vi "UserInterface_ZA.vi"(8 "error in":errorcluster, 9 "Zen Analytics":refnum<class "Zen Analytics.lvclass">, 11 "InitializationData":refnum<user-event>) -> (0 "error out":errorcluster)   [LabVIEW 2019, in "Zen Analytics.lvlib" / "Zen Analytics.lvclass"]
uses:
  Zen Analytics.lvclass
  Dependency/GraphReff.ctl
  <vilib>/Utility/miscctls.llb/LVRowAndColumnTypeDef.ctl
  <vilib>/Utility/miscctls.llb/LVBoundsTypeDef.ctl
panel:
  out "Bar graph":dbl[][](graph) caption="Defect Summary"
  out "Yeild Chart":picture
  out "Labels":picture
  out "Measurement-Summary -1":T1(graph)={"Start"=1, "index"=0, "Waveform Graph"=[]} caption="A Summary"
  out "Histogram Summary":T2(graph) caption="A Summary"
  in  "Select Measurement":u16(ring) items=["A", "C", "D"]
  out "Cp-CpkTable":string[][](table)=[["1.13", "1.14", "1.13", "1.16", "1.18"], ["1.14", "1.12", "1.12", "1.01", "1.02"], ["1.29", "1.26", "1.26", "1.03", "1.04"], ["0.10", "0.10", "0.13", "0.13", "0.11"], ["-0.05", "-0.10", "-0.17", "-0.07", "-0.22"]]
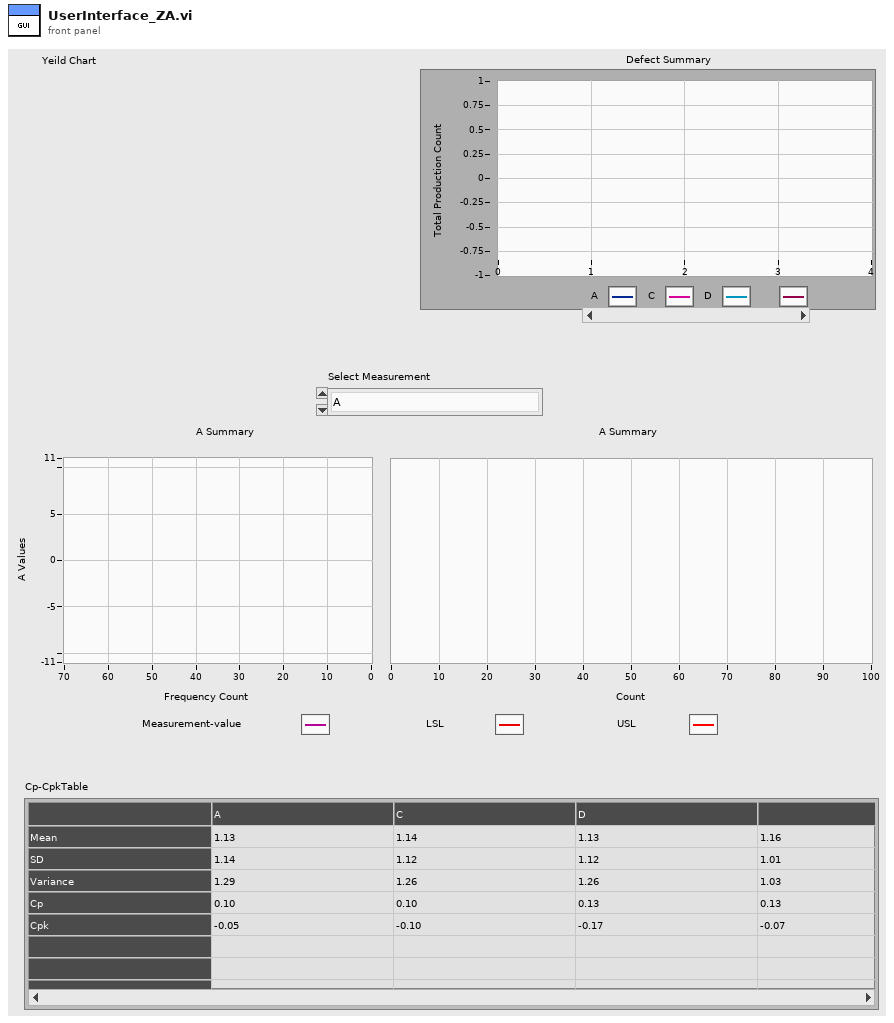
[diagram p1: front panel]
types:
  T1 = cluster{"Start":i32, "index":i32, "Waveform Graph":dbl[][]}
  T2 = cluster{"X Values":dbl[], "Best Gaussian Fit":dbl[]}[]
  T3 = typedef "LVRowAndColumnTypeDef.ctl" = cluster{"Row":i32, "Column":i32}
  T4 = typedef "LVBoundsTypeDef.ctl" = cluster{"Width":u32, "Height":u32}
  T5 = typedef "Zen Analytics.lvlib/Zen Analytics.lvclass/GraphReff.ctl" = cluster{"HistgramGraph-reff":refnum<vi>[], "BarGraph-reff":refnum<vi>[], "PieGraph-reff":refnum<vi>[], "Lable-reff":refnum<vi>[], "TrendGraph-reff":refnum<vi>[], "CpCpkTable":refnum<vi>}
  T6 = cluster{"ColumnNo":i32, "MeasurementData":cluster{"Measurement ID":i32, "Measurement Name":string, "Nominal Values":dbl, "LSL":dbl, "USL":dbl, "LCL":dbl, "UCL":dbl}[]}
  T7 = cluster{"Measurement ID":i32, "Measurement Name":string, "Nominal Values":dbl, "LSL":dbl, "USL":dbl, "LCL":dbl, "UCL":dbl}[]
  T8 = cluster{"Measurement-ID":i32[], "Measurement Names":string[], "NominalValues":dbl[], "LSL":dbl[], "USL":dbl[], "LCL":dbl[], "UCL":dbl[]}
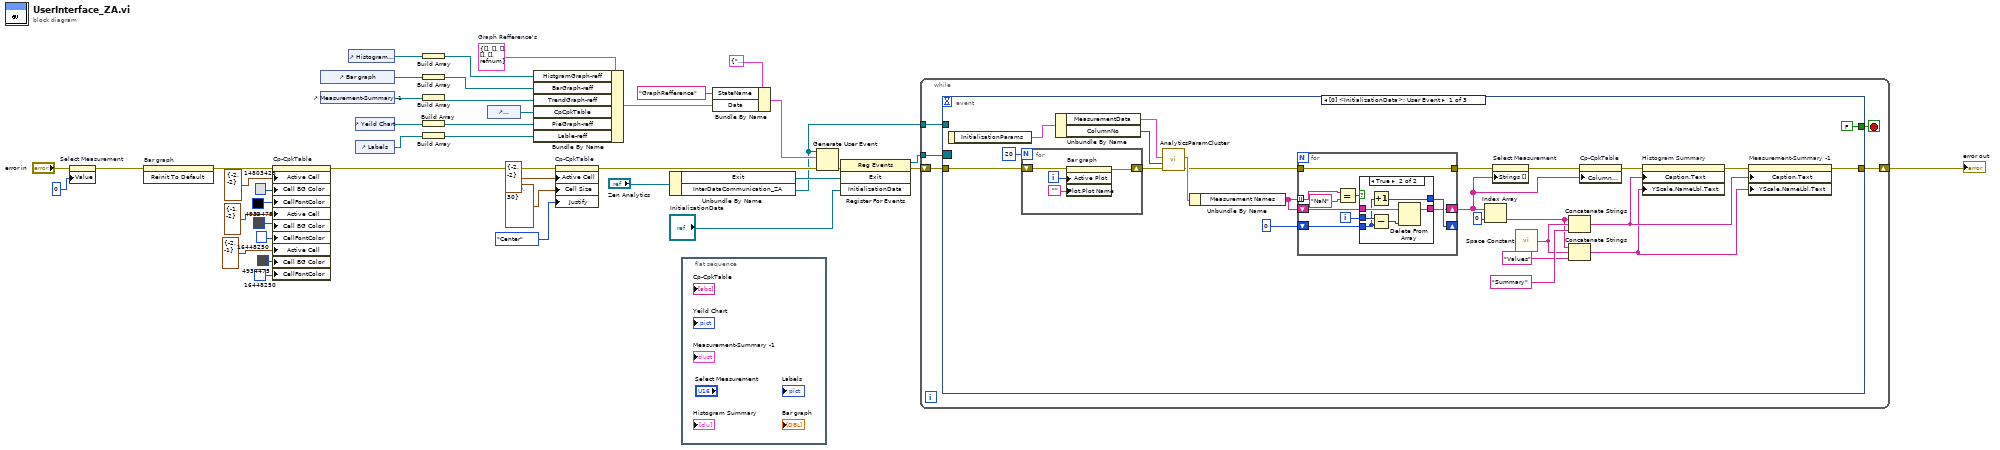
[diagram p0: block diagram]
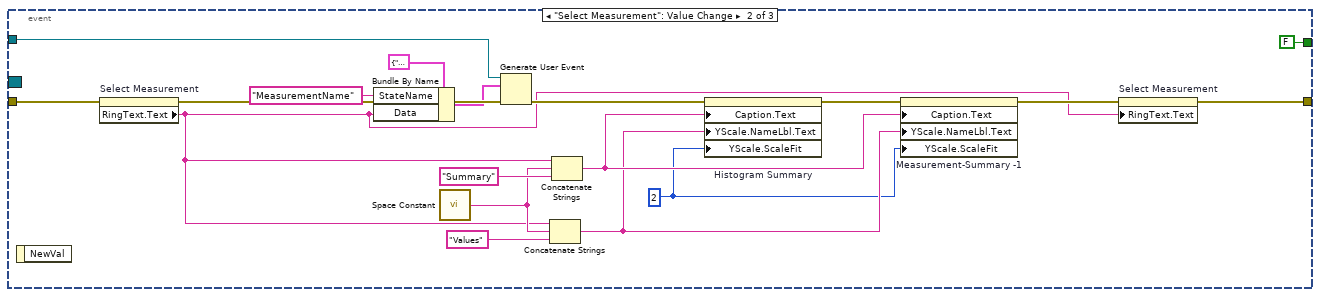
[diagram p3: hidden frame]
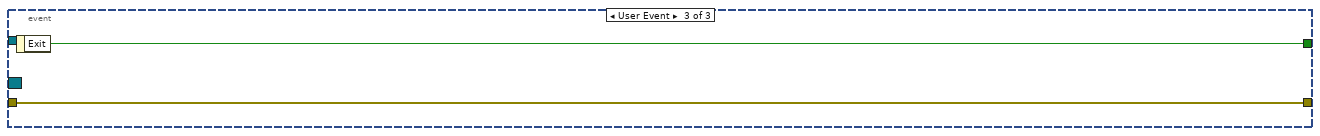
[diagram p4: hidden frame]
diagram:
  w39 = T5 {"HistgramGraph-reff"=[], "BarGraph-reff"=[], "PieGraph-reff"=[], "Lable-reff"=[], "TrendGraph-reff"=[], "CpCpkTable"=refnum}  # Graph Refference's
  n1 = property on="Select Measurement" class="Ring (strict)"(error in="error in", "Value"=0) -> (error out=w9:errorcluster)  [unwired: 1 in, 1 out]
  n2 = invoke on="Bar graph" class="WFGraph (strict)" method="Reinit To Default"(error in=w9) -> (error out=w8:errorcluster)  [unwired: 2 in, 2 out]
  n3 = property on="Cp-CpkTable" class="Tbl (strict)"(error in=w8, "Active Cell"=T3 {"Row"=-2, "Column"=-2} ("Active Cell:Active Cell"), "Cell BG Color"=u32 14803425, "CellFontColor"=u32 0, "Active Cell"=T3 {"Row"=-1, "Column"=-2} ("Active Cell:Active Cell"), "Cell BG Color"=u32 4934475, "CellFontColor"=u32 16448250, "Active Cell"=T3 {"Row"=-2, "Column"=-1} ("Active Cell:Active Cell"), "Cell BG Color"=u32 4934475, "CellFontColor"=u32 16448250) -> (error out=w24:errorcluster)  [unwired: 1 in, 1 out]
  n4 = control-ref of="Bar graph"() -> (w10:refnum<vi>)
  n5 = control-ref of="Measurement-Summary -1"() -> (w28:refnum<vi>)
  n6 = control-ref of="Histogram Summary"() -> (w27:refnum<vi>)
  n7 = control-ref of="Yeild Chart"() -> (w19:refnum<vi>)
  n8 = control-ref of="Labels"() -> (w20:refnum<vi>)
  n9 = Build Array(w27) -> (w38:refnum<vi>[])
  n10 = Build Array(w10) -> (w35:refnum<vi>[])
  n11 = Build Array(w28) -> (w37:refnum<vi>[])
  n12 = Build Array(w19) -> (w22:refnum<vi>[])
  n13 = Build Array(w20) -> (w21:refnum<vi>[])
  n14 = control-ref of="Cp-CpkTable"() -> (w36:refnum<vi>)
  n15 = Bundle By Name(cluster=w39, "HistgramGraph-reff"=w38, "BarGraph-reff"=w35, "TrendGraph-reff"=w37, "CpCpkTable"=w36, "PieGraph-reff"=w22, "Lable-reff"=w21) -> (w14:T5)
  n16 = property on="Cp-CpkTable" class="Tbl (strict)"(error in=w24, "Active Cell"=T3 {"Row"=-2, "Column"=-2} ("Active Cell:Active Cell"), "Cell Size"=T4 {"Width"=180, "Height"=30} ("Active Cell:Cell Size"), "Justify"=enum16{"Left", "Center", "Right"}."Center" ("Active Cell:Cell Justification")) -> (error out=w23:errorcluster)  [unwired: 1 in, 1 out]
  n17 = Unbundle By Name("Zen Analytics") -> ("Exit"=w31:refnum<user-event>, "InterDataCommunication_ZA"=w11:refnum<user-event>)
  n18 = flat-sequence {
    frame #0 {
    }
  }
  n19 = Bundle By Name(cluster=cluster{"StateName":string, "Data":variant} {"StateName"="", "Data"=variant} ("event data"), "StateName"="GraphRefference", "Data"=w14) -> (w15:cluster{"StateName":string, "Data":variant})
  n20 = Generate User Event(user event=w11, event data cluster=w15, error in=w23) -> (error out=w34:errorcluster)  [unwired: 1 in, 1 out]
  n21 = register-events(error in=w34, w31, "InitializationData") -> (reference out=w32:refnum<event-registration>, error out=w33:errorcluster)  [unwired: 1 in]
  n22 = while {
    shift-right: [w46] -> w25
    shift-left: w33 -> [w47]
    tunnel: w32 -> [w45]
    tunnel: w11 -> [w43]
    stop <- w44 stop-if-true
    n23 = event shown="[0] <InitializationData>: User Event" {
      selector: w45 -> [_ _ _]
      dyn-events: _ -> [_ _ _]
      timeout: _ -> [_ _ _]
      tunnel: w47 -> [w50 w110 w111]
      tunnel: [w56 w94 w111] -> w46
      tunnel: [FALSE ("Exit") FALSE ("Exit") w112] -> w44
      tunnel: w43 -> [_ w102 _]
      event User Event {
        n24 = event-data() -> ("InitializationParams"=w54:T6)  [unwired: 1 in]
        n25 = for {
          N: 20 -> [_]
          shift-right: [w72] -> w49
          shift-left: w50 -> [w73]
          i -> [w75]
          n26 = property on="Bar graph" class="WFGraph (strict)"(error in=w73, "Active Plot"=w75, "Plot.Plot Name"="") -> (error out=w72:errorcluster)  [unwired: 1 in, 1 out]
        }
        n27 = Unbundle By Name(w54) -> ("MeasurementData"=w53:T7, "ColumnNo"=w52:i32)
        n28 = call "AnalyticsParamCluster.vi"("error in (no error)"=w49, "Number of columns"=w52, "MeasurementData"=w53) -> ("error out"=w60:errorcluster, "Initialization Data"=w71:T8)  [unwired: 6 in, 1 out]
        n29 = Unbundle By Name(w71) -> ("Measurement Names"=w63:string[])
        n30 = for {
          tunnel: w63 -> [w78] mode=indexing
          shift-right: [w83] -> _
          shift-left: 0 -> [w84]
          shift-right: [w80] -> w57
          shift-left: w63 -> [w81]
          tunnel: [w76] -> w55
          tunnel: w60 -> [w76]
          i -> [w82]
          n31 = Equal?(x=w78, y="NaN") -> (x = y?=w77:bool)
          n32 = case shown="True" w77 {
            tunnel: w81 -> [w85 w92]
            tunnel: w84 -> [w86 w87]
            tunnel: [w86 w90] -> w83
            tunnel: [w85 w91] -> w80
            tunnel: w82 -> [_ w88]
            frame False {
            }
            frame True {
              n33 = Increment(x=w87) -> (x+1=w90:i32)
              n34 = Subtract(x=w88, y=w87) -> (x-y=w89:i32)
              n35 = Delete From Array(array=w92, index=w89) -> (array with subset deleted=w91:string[])  [unwired: 1 in, 1 out]
            }
          }
        }
        n36 = Index Array(array=w57, index=0) -> (element=w59:string)
        n37 = property on="Select Measurement" class="Ring (strict)"(error in=w55, "Strings []"=w57) -> (error out=w67:errorcluster)  [unwired: 1 in, 1 out]
        n38 = call <vilib>:"Space Constant.vi"() -> ("String"=w65:string)
        n39 = Concatenate Strings(w59, w65, "Summary" ("string")) -> (w68:string)
        n40 = Concatenate Strings(w59, w65, "Values" ("string")) -> (w58:string)
        n41 = property on="Cp-CpkTable" class="Tbl (strict)"(error in=w67, "Column Headers[]"=w57) -> (error out=w66:errorcluster)  [unwired: 1 in, 1 out]
        n42 = property on="Histogram Summary" class="XYGraph (strict)"(error in=w66, "Caption.Text"=w68, "YScale.NameLbl.Text"=w58) -> (error out=w69:errorcluster)  [unwired: 1 in, 1 out]
        n43 = property on="Measurement-Summary -1" class="WFGraph (strict)"(error in=w69, "Caption.Text"=w68, "YScale.NameLbl.Text"=w58) -> (error out=w56:errorcluster)  [unwired: 1 in, 1 out]
      }
      event "Select Measurement": Value Change {
        w96 = u8 2 ("Y Scale.Scale Fit")
        n44 = event-data() -> ()  [unwired: 1 in, 1 out]
        n45 = property on="Select Measurement" class="Ring (strict)"(error in=w110) -> (error out=w109:errorcluster, "RingText.Text"=w93:string)  [unwired: 1 in, 1 out]
        n46 = Bundle By Name(cluster=cluster{"StateName":string, "Data":variant} {"StateName"="", "Data"=variant} ("event data"), "StateName"="MeasurementName", "Data"=w93) -> (w99:cluster{"StateName":string, "Data":variant})
        n47 = call <vilib>:"Space Constant.vi"() -> ("String"=w98:string)
        n48 = Generate User Event(user event=w102, event data cluster=w99, error in=w109) -> (error out=w107:errorcluster)  [unwired: 1 in, 1 out]
        n49 = Concatenate Strings(w93, w98, "Values" ("string")) -> (w103:string)
        n50 = Concatenate Strings(w93, w98, "Summary" ("string")) -> (w105:string)
        n51 = property on="Histogram Summary" class="XYGraph (strict)"(error in=w107, "Caption.Text"=w105, "YScale.NameLbl.Text"=w103, "YScale.ScaleFit"=w96) -> (error out=w106:errorcluster)  [unwired: 1 in, 1 out]
        n52 = property on="Measurement-Summary -1" class="WFGraph (strict)"(error in=w106, "Caption.Text"=w105, "YScale.NameLbl.Text"=w103, "YScale.ScaleFit"=w96) -> (error out=w95:errorcluster)  [unwired: 1 in, 1 out]
        n53 = property on="Select Measurement" class="Ring (strict)"(error in=w95, "RingText.Text"=w93) -> (error out=w94:errorcluster)  [unwired: 1 in, 1 out]
      }
      event User Event {
        n54 = event-data() -> ("Exit"=w112:bool)  [unwired: 1 in]
      }
    }
  }
  "error out" <- w25
